vi "Rename.vi"(8 "error in (no error)":errorcluster, 10 "name":string, 11 "variant in":variant) -> (0 "error out":errorcluster, 3 "variant out":variant)   [LabVIEW 2019, in "JSON.lvlib"]
doc: "Renames the varient in.\n\nCreated by: Ryan Pacini"
uses:
  JSON.lvlib
  <vilib>/Utility/Data Type/NI_Data Type.lvlib
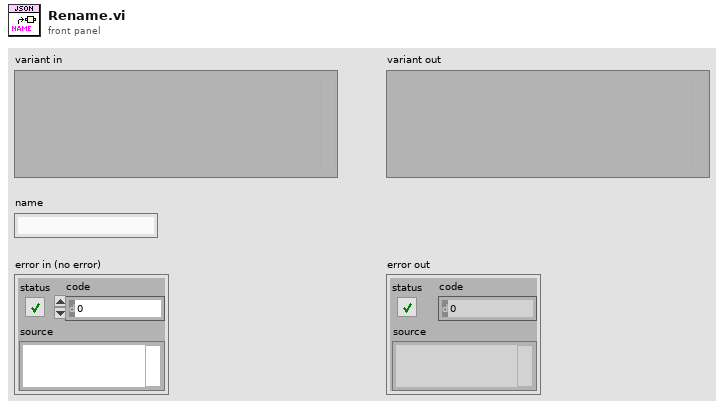
[diagram p1: front panel]
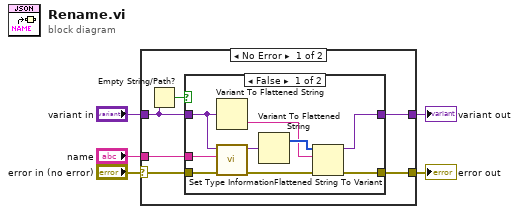
[diagram p0: block diagram]
diagram:
  n1 = case shown="No Error" "error in (no error)" {
    selector: "error in (no error)" -> [w8 w24]
    tunnel: [w9 w24] -> w5
    tunnel: [w11 w23] -> w3
    tunnel: "variant in" -> [w7 w23]
    tunnel: "name" -> [w10 _]
    frame No Error {
      n2 = Empty String/Path?(string/path=w7) -> (empty?=w6:bool)
      n3 = case shown="False" w6 {
        tunnel: [w20 w22] -> w11
        tunnel: w10 -> [w19 _]
        tunnel: [w18 w21] -> w9
        tunnel: w8 -> [w17 w21]
        tunnel: w7 -> [w12 w22]
        frame False {
          n4 = Variant To Flattened String(Variant=w12) -> (data string=w13:string)  [unwired: 1 out]
          n5 = call <vilib>:"Set Type Information.vi"("error in (no error)"=w17, "Name"=w19, "Variant in"=w12) -> ("error out"=w16:errorcluster, "Variant out"=w15:variant)  [unwired: 7 in]
          n6 = Variant To Flattened String(Variant=w15) -> (1:w14:i16[])  [unwired: 1 out]
          n7 = Flattened String To Variant(4:w16, 6:w13, 7:w14) -> (0:w18:errorcluster, 3:w20:variant)
        }
        frame True {
        }
      }
    }
    frame Error {
    }
  }
  "error out" <- w5
  "variant out" <- w3
